vi "Dynamic Bit Depth Encoding x8 (SubVI).vi"(0 "Pixel Data In":u64, 5 "Pixel In Valid?":bool=TRUE, 8 "Block Size x2":u16=8, 10 "Block Size":u16=8, 12 "Image Width":u16=512) -> (14 "Bit Depth":u8, 15 "Minimum":u8, 16 "BD-Min Valid?":bool, 17 "Pixel Sync":bool, 18 "Data Out":u64, 19 "Data Valid?":bool)   [LabVIEW 2015]
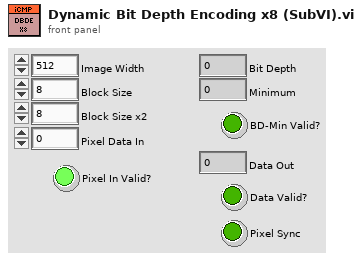
[diagram p1: front panel]
types:
  T1 = cluster{"Numeric Control":u8, "Numeric Control":u8, "Numeric Control":u8, "Numeric Control":u8, "Numeric Control":u8, "Numeric Control":u8, "Numeric Control":u8, "Numeric Control":u8}
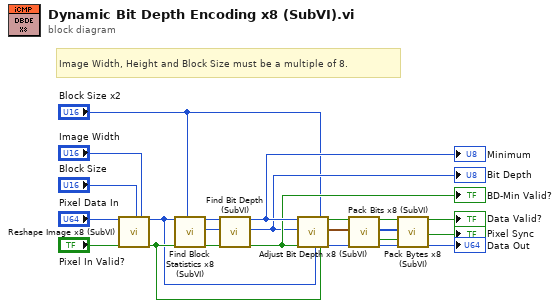
[diagram p0: block diagram]
diagram:
  # "Image Width, Height and Block Size must be a multiple of 8."
  n1 = call "Reshape Image x8 (SubVI).vi"("Pixel Data In"="Pixel Data In", "Pixel In Valid?"="Pixel In Valid?", "Block Size"="Block Size", "Image Width"="Image Width") -> ("Pixel Data Out"=w11:u64, "Pixel Out Valid?"=w12:bool)  [unwired: 14 in]
  n2 = call "Find Block Statistics x8 (SubVI).vi"("Pixel Data"=w11, "Pixel Valid?"=w12, "Block Size x2"="Block Size x2") -> ("Maximum"=w13:u8, "Minimum"=w14:u8, "Result Valid?"=w15:bool)  [unwired: 14 in]
  n3 = call "Find Bit Depth (SubVI).vi"("Maximum"=w13, "Minimum (In)"=w14, "Input Valid?"=w15) -> ("Minimum (Out)"=w19:u8, "Bit Depth"=w17:u8, "Output Valid?"=w18:bool)  [unwired: 14 in]
  "BD-Min Valid?" <- w18
  "Minimum" <- w19
  "Bit Depth" <- w17
  n4 = call "Adjust Bit Depth x8 (SubVI).vi"("Minimum"=w19, "Bit Depth"=w17, "Stat. Valid?"=w18, "Pixel Data"=w11, "Block Size x2"="Block Size x2", "Pixel Valid?"=w12) -> ("Output Valid?"=w9:bool, "Data Out"=w8:T1, "Bid Depth Out"=w16:u8)  [unwired: 11 in]
  n5 = call "Pack Bits x8 (SubVI).vi"("Input Valid?"=w9, "Data In"=w8, "Bit Depth"=w16) -> ("Output Valid?"=w7:bool, "Data Out"=w5:u8[], "Pixel Sync"=w1:bool, "N Bytes"=w6:u8)  [unwired: 13 in]
  n6 = call "Pack Bytes x8 (SubVI).vi"("Input Valid?"=w7, "Data In"=w5, "Pixel Sync In"=w1, "N Bytes"=w6) -> ("Output Valid?"=→"Data Valid?":bool, "Pixel Sync Out"=→"Pixel Sync":bool, "Data Out"=→"Data Out":u64)  [unwired: 13 in]
